vi "advanced edge detection clamp with angle.vi"(0 "Refnum in":T8, 1 "Search Direction":i32, 3 "Staright Edges of Co-ordinate":T6, 4 "Measurement":T5, 5 "error in (no error)":errorcluster, 6 "Small ROI":T7, 8 "Edge Options":T3={"Edge Polarity"=0, "Kernel Size"=3, "Width"=3, "Minimum Edge Strength"=10.0, "Interpolation Type"=enum."Bilinear Fixed", "Data Processing Method"=enum."Average"} {"Edge Polarity" items=["All Edges", "Rising Edges", "Falling Edges"]; "Minimum Edge Strength" format="%.2f"; "Width" step=2; "Kernel Size" step=2}, 9 "Line Options":T1={"Number of Lines"=1, "Type"=enum."Best Edge Projection", "Min. Score"=10.0, "Max. Score"=1000.0, "Orientation"=0.0, "Angle Range"=10.0, "Angle Tolerance"=1.0, "Step Size"=3, "Min. SNR (db)"=0.0, "Min. Points (%)"=25.0, "Hough Iterations"=5} {"Min. Points (%)" min=0.0 max=100.0; "Min. SNR (db)" min=0.0; "Max. Score" min=0.0 max=1024.0; "Min. Score" min=0.0 max=1024.0 step=1.0}, 10 "ROI 2":T7) -> (14 "Refnum out":T8, 15 "ROI Descriptor":T9 {"Contours"."Type" items=["No Selection", "Point", "Line", "Rectangle", "Oval", "Polygon", "Freehand Region", "Annulus", "Unused2", "Unused3", "Broken Line", "Freehand Line", "Rotated Rectangle"]}, 16 "Edge Points-Array":cluster{"X":sgl, "Y":sgl}[][](array[cluster]), 19 "error out":errorcluster)   [LabVIEW 2014]
uses:
  <vilib>/vision/Image Controls.llb/IMAQ Image.ctl
  <vilib>/vision/Measure.llb/Edge Options.ctl
  <vilib>/vision/Measure.llb/Edge Polarity.ctl
  <vilib>/vision/Measure.llb/Straight Edge Options.ctl
  <vilib>/vision/Measure.llb/Straight Edge Process.ctl
  <vilib>/vision/NI_Vision_Development_Module.lvlib
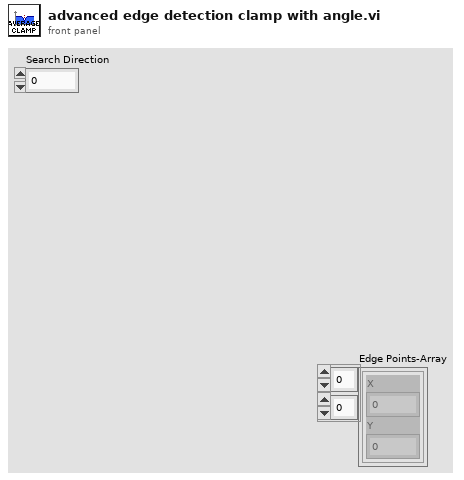
[diagram p1: front panel]
types:
  T1 = typedef "Straight Edge Options.ctl" = cluster{"Number of Lines":i32, "Type":T2, "Min. Score":dbl, "Max. Score":dbl, "Orientation":dbl, "Angle Range":dbl, "Angle Tolerance":dbl, "Step Size":u32, "Min. SNR (db)":dbl, "Min. Points (%)":dbl, "Hough Iterations":i32}
  T2 = typedef "Straight Edge Process.ctl" = enum32{"First Edge Rake", "Best Edge Rake", "Hough Edge Rake", "First Edge Projection", "Best Edge Projection"}
  T3 = typedef "Edge Options.ctl" = cluster{"Edge Polarity":T4, "Kernel Size":u32, "Width":u32, "Minimum Edge Strength":sgl, "Interpolation Type":enum32{"Zero Order", "Bilinear", "Quadratic", "Cubic", "Bilinear Fixed"}, "Data Processing Method":enum32{"Average", "Median"}}
  T4 = typedef "Edge Polarity.ctl" = u32
  T5 = cluster{"Origin":cluster{"X":sgl, "Y":sgl}, "Angle (deg)":sgl, "Axis Reference":u32}
  T6 = cluster{"Point1 (Pixels)":cluster{"X":sgl, "Y":sgl}, "Point2 (Pixels)":cluster{"X":sgl, "Y":sgl}}
  T7 = cluster{"Global Rectangle":i32[], "Contours":cluster{"Contour Type":u32, "ROI Type":u32, "Points":i32[]}[]}
  T8 = typedef "IMAQ Image.ctl" = refnum<image>
  T9 = typedef "ROI Descriptor" = cluster{"Global Rectangle":i32[], "Contours":cluster{"ID":enum32{"External", "Internal"}, "Type":u32, "Coordinates":i32[]}[]}
  T10 = typedef "IMAQ Rectangle" = cluster{"Left":i32, "Top":i32, "Right":i32, "Bottom":i32, "Rotation":dbl}
  T11 = cluster{"Point1 (Pixels)":cluster{"X":sgl, "Y":sgl}, "Point2 (Pixels)":cluster{"X":sgl, "Y":sgl}, "Point1 (Real-World)":cluster{"X":sgl, "Y":sgl}, "Point2 (Real-World)":cluster{"X":sgl, "Y":sgl}, "Angle (Pixel)":dbl, "Angle (Real-World)":dbl, "Score":dbl, "Straightness":dbl, "Average SNR (db)":dbl, "Calibration Valid":bool}[]
  T12 = cluster{"Point1 (Pixels)":cluster{"X":sgl, "Y":sgl}, "Point2 (Pixels)":cluster{"X":sgl, "Y":sgl}, "Point1 (Real-World)":cluster{"X":sgl, "Y":sgl}, "Point2 (Real-World)":cluster{"X":sgl, "Y":sgl}, "Angle (Pixel)":dbl, "Angle (Real-World)":dbl, "Score":dbl, "Straightness":dbl, "Average SNR (db)":dbl, "Calibration Valid":bool}
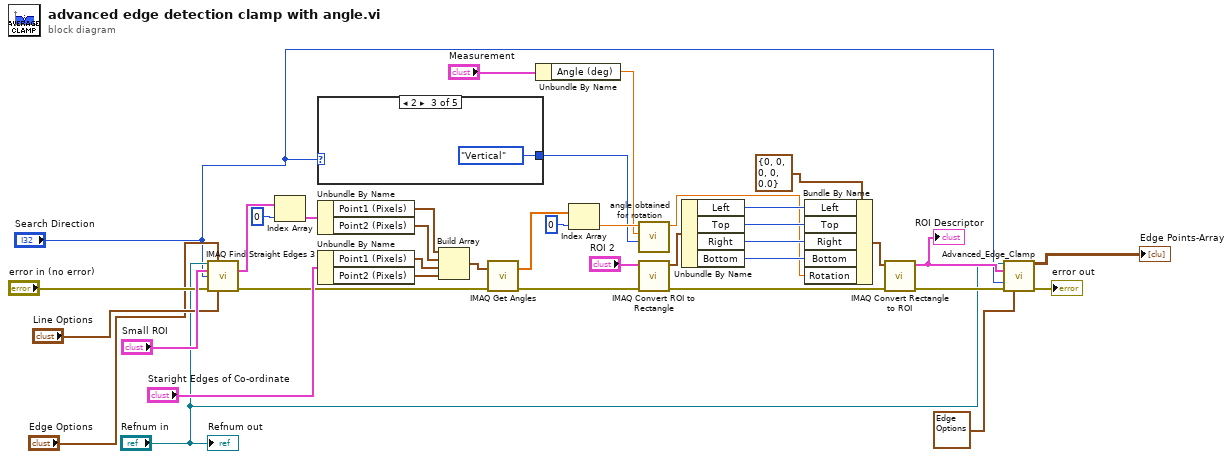
[diagram p0: block diagram]
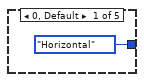
[diagram p2: hidden frame]
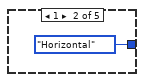
[diagram p3: hidden frame]
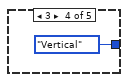
[diagram p4: hidden frame]
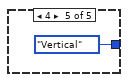
[diagram p5: hidden frame]
diagram:
  n1 = call "IMAQ Find Straight Edges 3"("Image"="Refnum in", "Edge Options"="Edge Options", "ROI Descriptor"="Small ROI", "Search Direction"="Search Direction", "error in (no error)"="error in (no error)", "Line Options"="Line Options") -> ("Straight Edges"=w1:T11, "error out"=w11:errorcluster)  [unwired: 5 in, 3 out]
  n2 = Index Array(array=w1, index=0) -> (element=w38:T12)
  n3 = case shown="2" "Search Direction" {
    tunnel: [enum16{"Horizontal", "Vertical"}."Horizontal" ("Search Direction") enum16{"Horizontal", "Vertical"}."Horizontal" ("Search Direction") enum16{"Horizontal", "Vertical"}."Vertical" ("Search Direction") enum16{"Horizontal", "Vertical"}."Vertical" ("Search Direction") enum16{"Horizontal", "Vertical"}."Vertical" ("Search Direction")] -> w3
    frame 0, Default {
    }
    frame 1 {
    }
    frame 2 {
    }
    frame 3 {
    }
    frame 4 {
    }
  }
  n4 = Unbundle By Name(w38) -> ("Point1 (Pixels)"=w32:cluster{"X":sgl, "Y":sgl}, "Point2 (Pixels)"=w33:cluster{"X":sgl, "Y":sgl})
  n5 = Unbundle By Name("Staright Edges of Co-ordinate") -> ("Point1 (Pixels)"=w18:cluster{"X":sgl, "Y":sgl}, "Point2 (Pixels)"=w19:cluster{"X":sgl, "Y":sgl})
  n6 = Build Array(w32, w33, w18, w19) -> (w20:cluster{"X":sgl, "Y":sgl}[])
  n7 = call "IMAQ Get Angles"("error in (no error)"=w11, "Points"=w20) -> ("error out"=w23:errorcluster, "Angles (deg)"=w21:sgl[])  [unwired: 3 in, 1 out]
  n8 = Unbundle By Name("Measurement") -> ("Angle (deg)"=w15:sgl)
  n9 = Index Array(array=w21, index=0) -> (element=w30:sgl)
  n10 = call "angle obtained for rotation.vi"("Search Direction"=w3, "Angle (deg) System"=w15, "Angle (deg) Obtained"=w30) -> ("Total Rotation"=w13:dbl)  [unwired: 8 in]
  n11 = call "IMAQ Convert ROI to Rectangle"("error in (no error)"=w23, "ROI Descriptor"="ROI 2") -> ("error out"=w31:errorcluster, "Rectangle"=w24:T10)  [unwired: 7 in]
  n12 = Unbundle By Name(w24) -> ("Left"=w26:i32, "Top"=w27:i32, "Right"=w28:i32, "Bottom"=w29:i32)
  n13 = Bundle By Name(cluster=T10 {"Left"=0, "Top"=0, "Right"=0, "Bottom"=0, "Rotation"=0.0} ("Rectangle"), "Left"=w26, "Top"=w27, "Right"=w28, "Bottom"=w29, "Rotation"=w13) -> (w35:T10)
  n14 = call "IMAQ Convert Rectangle to ROI"("error in (no error)"=w31, "Rectangle"=w35) -> ("error out"=w7:errorcluster, "ROI Descriptor"=w9:T9)  [unwired: 7 in]
  "ROI Descriptor" <- w9
  n15 = call "Advanced_Edge_Clamp.vi"("Image"="Refnum in", "ROI Descriptor"=w9, "Search Direction"="Search Direction", "error in (no error)"=w7, "Edge Options"=T3 {"Edge Polarity"=0, "Kernel Size"=7, "Width"=5, "Minimum Edge Strength"=40.0, "Interpolation Type"=enum."Bilinear", "Data Processing Method"=enum."Average"}) -> ("Edge Points-Array"=→"Edge Points-Array":cluster{"X":sgl, "Y":sgl}[][], "error out"=→"error out":errorcluster)  [unwired: 9 in]
  "Refnum out" <- "Refnum in"
